vi "Set remote state.vi"(8 "error in":errorcluster, 9 "Override instr. error (true)":bool=TRUE, 10 "Remote state":u16(ring)=2 items=["Local", "Remote", "Default"], 11 "VISA resource name":refnum<visa-resource-name>) -> (0 "error out":errorcluster, 3 "VISA resource name out":refnum<visa-resource-name>)   [LabVIEW 2020, in "Datron D4xxx.lvlib"]
doc: "This VI sets instrument remote mode to desired value. If you choose \"Default\" remote will be set to state which was previously defined by \"Set default remote state\" VI.\nInput \"override instrument error\" means that VI will try to set remote mode even if \"error in\" contains non-VISA error."
uses:
  Datron D4xxx.lvlib
  <vilib>/Instr/_visa.llb/VISA GPIB Control REN Mode.ctl
  Private/vars.vi
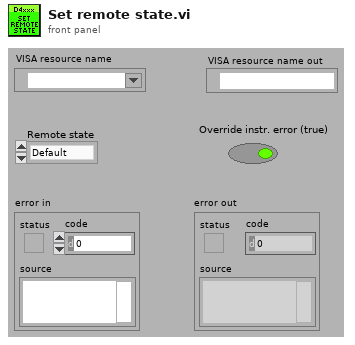
[diagram p1: front panel]
types:
  T1 = typedef "VISA GPIB Control REN Mode.ctl" = u16
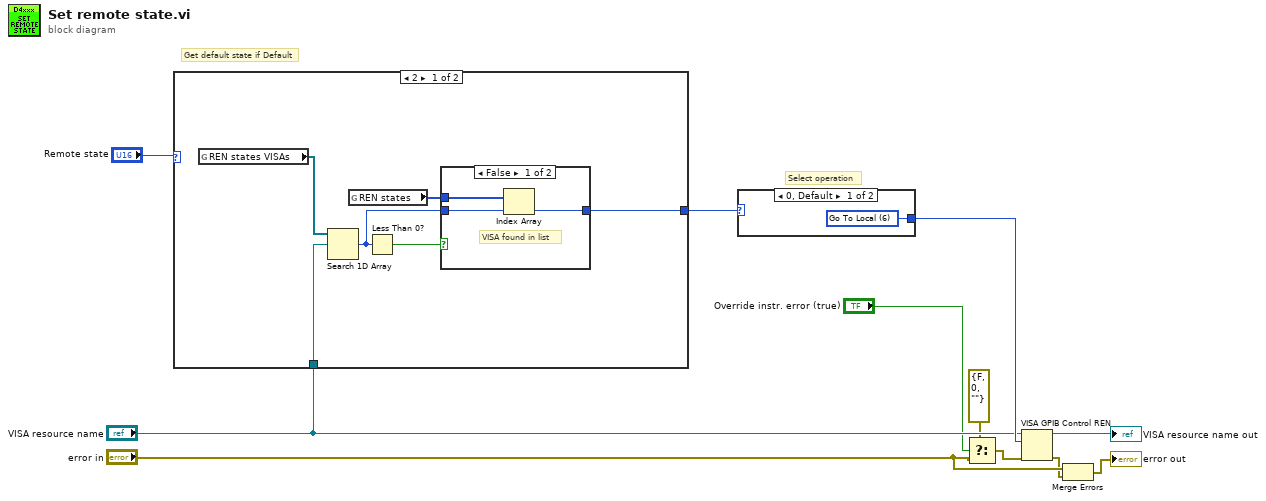
[diagram p0: block diagram]
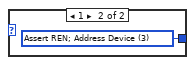
[diagram p2: hidden frame]
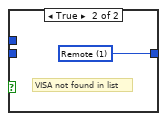
[diagram p3: hidden frame]
diagram:
  # "Select operation"
  # "Get default state if Default"
  n1 = case shown="2" "Remote state" {
    selector: "Remote state" -> [_ w22]
    tunnel: [w12 w22] -> w10
    tunnel: "VISA resource name" -> [w16 _]
    frame 2 {
      n2 = global read "vars.vi" "REN states VISAs"() -> (w17:refnum<visa-resource-name>[])
      n3 = Search 1D Array(1D array=w17, element=w16) -> (index of element=w13:i32)  [unwired: 1 in]
      n4 = global read "vars.vi" "REN states"() -> (w14:u16[])
      n5 = Less Than 0?(x=w13) -> (x < 0?=w15:bool)
      n6 = case shown="False" w15 {
        tunnel: w14 -> [w20 _]
        tunnel: w13 -> [w19 _]
        tunnel: [w18 w21] -> w12
        frame False {
          # "VISA found in list"
          n7 = Index Array(array=w20, index=w19) -> (element=w18:u16)
        }
        frame True {
          w21 = u16 1 items=["Local", "Remote", "Default"] ("Remote state")
          # "VISA not found in list"
        }
      }
    }
    frame Default {
    }
  }
  n8 = case shown="0, Default" w10 {
    tunnel: [w23 w24] -> w9
    frame 0, Default {
      w23 = T1 6 items=["Deassert REN", "Assert REN", "Go To Local; Deassert REN ", "Assert REN; Address Device", "Local Lockout (Addressed Devices)", "Local Lockout (This Device)", "Go To Local"] ("Mode")
    }
    frame 1 {
      w24 = T1 3 items=["Deassert REN", "Assert REN", "Go To Local; Deassert REN ", "Assert REN; Address Device", "Local Lockout (Addressed Devices)", "Local Lockout (This Device)", "Go To Local"] ("Mode")
    }
  }
  n9 = Select(t=errorcluster {"status"=FALSE, "code"=0, "source"=""}, s="Override instr. error (true)", f="error in") -> (s? t:f=w5:errorcluster)
  n10 = VISA GPIB Control REN(8:w5, 10:w9, 11:"VISA resource name") -> (0:w1:errorcluster, 3:→"VISA resource name out":refnum<visa-resource-name>)
  n11 = Merge Errors("error in", w1) -> (→"error out":errorcluster)
